vi "TelemetryServer_QueuePump.vi"(3 "Telemetry queues in":refnum<queue>[](array[refnum]), 9 "Error out":errorcluster caption="error in (no error)") -> (0 "Telemetry queues out":refnum<queue>[](array[refnum]), 2 "Waveforms out":waveform(dbl)[](array[waveform]), 6 "error in":errorcluster caption="error out")   [LabVIEW 2009]
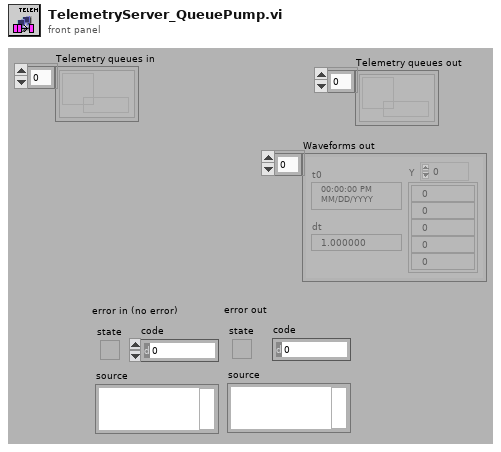
[diagram p1: front panel]
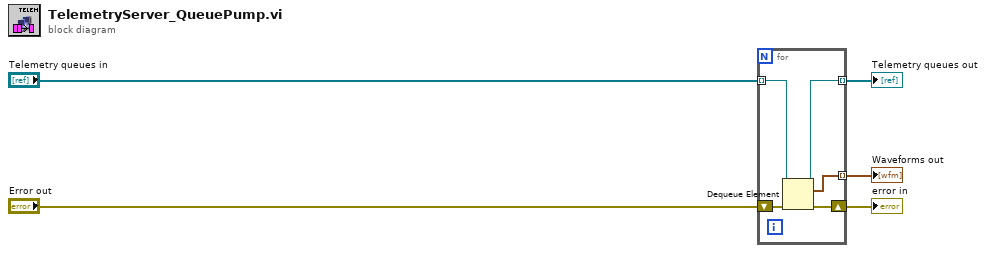
[diagram p0: block diagram]
diagram:
  n1 = for {
    tunnel: "Telemetry queues in" -> [w9] mode=indexing
    tunnel: [w7] -> w5 mode=indexing
    shift-right: [w8] -> w4
    shift-left: "Error out" -> [w10]
    tunnel: [w6] -> w3 mode=indexing
    n2 = Dequeue Element(queue=w9, error in (no error)=w10) -> (queue out=w7:refnum<queue>, element=w6:waveform(dbl), error out=w8:errorcluster)  [unwired: 2 out]
  }
  "Waveforms out" <- w3
  "error in" <- w4
  "Telemetry queues out" <- w5
